vi "backgroundSubstraction.vi"(8 "inputValid":bool=TRUE, 11 "input":cluster{"index":u16, "data":i16}) -> (0 "outptValid":bool, 2 "background":i16, 3 "output":cluster{"index":u16, "data":i16})   [LabVIEW 2016]
uses:
  <vilib>/rvi/Memory/Memory_Emulation/nirvimemoryFastEmulation.vi
  <vilib>/rvi/Memory/Memory_Emulation/nirvimemoryEmulation.vi
  <vilib>/rvi/Emulation/niFpgaEmulationIsFPGAContextNoSignature.vi
  <vilib>/rvi/DataTransferAndStorage/Container/Common/niFpgaContainerGetUniqueNameForEmu.vi
  <vilib>/rvi/Emulation/niFpgaProcessEmulError.vi
  <vilib>/rvi/Emulation/niFpgaSctlEmulationGetInTimedLoop.vi
  <vilib>/rvi/errors/nirviReportUnexpectedCaseInternalError (U32).vi
  <vilib>/rvi/DataTransferAndStorage/Container/XNode/niFpgaContainer.xnode
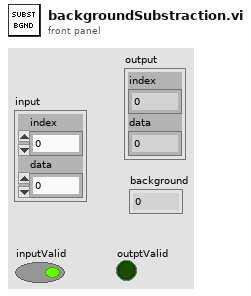
[diagram p1: front panel]
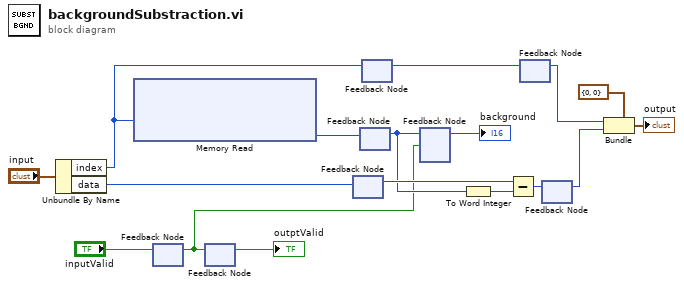
[diagram p0: block diagram]
diagram:
  n1 = Unbundle By Name("input") -> ("index"=w12:u16, "data"=w16:i16)
  n2 = xnode ("Memory Read")("Address"=w12) -> ("Data"=w17:i16)  [unwired: 1 in, 1 out]
  n3 = feedback #1() -> (w1:bool)  [unwired: 1 in]
  n4 = feedback-in #1("inputValid") -> ()
  n5 = feedback #2() -> (→"outptValid":bool)  [unwired: 1 in]
  n6 = feedback-in #2(w1) -> ()
  n7 = feedback #3() -> (w11:i16)  [unwired: 1 in]
  n8 = feedback-in #3(w16) -> ()
  n9 = feedback #4() -> (w7:i16)  [unwired: 1 in]
  n10 = feedback-in #4(w17) -> ()
  n11 = feedback #5() -> (w14:u16)  [unwired: 1 in]
  n12 = feedback-in #5(w12) -> ()
  n13 = feedback-in #6(w7, w1) -> ()
  n14 = feedback #6() -> (→"background":i16)  [unwired: 1 in]
  n15 = To Word Integer(number=w7) -> (16bit integer=w13:i16)
  n16 = Subtract(x=w11, y=w13) -> (x-y=w15:i16)
  n17 = feedback #7() -> (w9:u16)  [unwired: 1 in]
  n18 = feedback-in #7(w14) -> ()
  n19 = feedback #8() -> (w8:i16)  [unwired: 1 in]
  n20 = feedback-in #8(w15) -> ()
  n21 = Bundle(cluster=cluster{"index":u16, "data":i16} {"index"=0, "data"=0} ("dataPair"), "index"=w9, "data"=w8) -> (→"output":cluster{"index":u16, "data":i16})
